vi "Read Timing.vi"(8 "error in (no error)":errorcluster, 11 "Sim Display Console Actor in":refnum<class "Sim Display Console Actor.lvclass">) -> (0 "error out":errorcluster, 3 "Sim Display Console Actor out":refnum<class "Sim Display Console Actor.lvclass">)   [LabVIEW 2019, in "Sim Display Console Actor.lvlib" / "Sim Display Console Actor.lvclass"]
uses:
  Sim Display Console Actor.lvclass
  <vilib>/ActorFramework/Actor/Actor.lvclass
  Elevator Controller/Elevator Controller Messages/Get Elevator Location Msg/Get Elevator Location Msg.lvclass
  C:/Workspace/CLA/Elevator AF 3rd/Display Console Actor/Display Console Actor/Display Console Actor.lvclass
  C:/Program Files (x86)/National Instruments/LabVIEW 2019/vi.lib/ActorFramework/Actor/Actor.lvclass
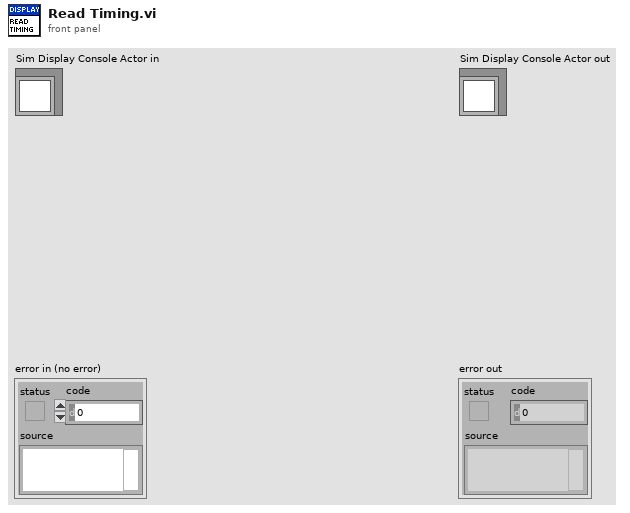
[diagram p1: front panel]
types:
  T1 = typedef "Sim Display Console Actor.lvlib/Sim Display Console Actor.lvclass/Floors -Enum.ctl" = enum16{"1st Floor", "2nd Floor", "3rd Floor", "4th Floor"}
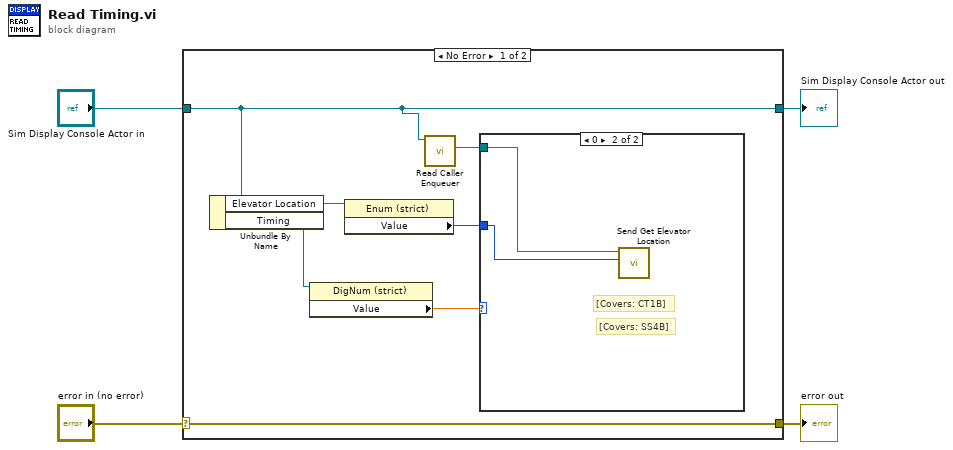
[diagram p0: block diagram]
diagram:
  n1 = case shown="No Error" "error in (no error)" {
    selector: "error in (no error)" -> [w11 w15]
    tunnel: [w11 w15] -> w3
    tunnel: [w6 w14] -> w1
    tunnel: "Sim Display Console Actor in" -> [w6 w14]
    frame No Error {
      n2 = Unbundle By Name(w6) -> ("Elevator Location"=w8:refnum<vi>, "Timing"=w10:refnum<vi>)
      n3 = property class="DigNum (strict)"(reference=w10) -> ("Value"=w9:dbl)  [unwired: 1 in, 2 out]
      n4 = property class="Enum (strict)"(reference=w8) -> ("Value"=w7:T1)  [unwired: 1 in, 2 out]
      n5 = call <vilib>:"Read Caller Enqueuer.vi"("Actor"=w6) -> ("Caller Enqueuer"=w5:refnum<class "Message Enqueuer.lvclass">)  [unwired: 10 in]
      n6 = case shown="0" w9 {
        tunnel: w7 -> [_ w12]
        tunnel: w5 -> [_ w13]
        frame 0 {
        }
        frame 0 {
          # "[Covers: SS4B]"
          # "[Covers: CT1B]"
          n7 = call "Send Get Elevator Location.vi"("Elevator Location"=w12, "Message Enqueuer"=w13) -> ()  [unwired: 8 in, 2 out]
        }
      }
    }
    frame Error {
    }
  }
  "error out" <- w3
  "Sim Display Console Actor out" <- w1
